vi "Get All API Interface Info.vi"(8 "error in (no error)":errorcluster, 11 "CSM-Helper in":refnum<class "CSM-Helper.lvclass">) -> (0 "error out":errorcluster, 2 "Array":cluster{string, "Array":T1[], "Response":T1[]}[](array[cluster]), 3 "CSM-Helper out":refnum<class "CSM-Helper.lvclass">)   [LabVIEW 2017, in "CSM-Helper.lvclass"]
doc: "### Get All API Interface Info.vi\n\n-- <b>Controls</b> --\n- <b>CSM-Helper in</b>: CSMHelper input\n\n-- <b>Indicators</b> --\n- <b>Array</b>:\n- <b>CSM-Helper out</b>: CSMHelper output"
uses:
  CSM-Helper.lvclass
  Typedef/Def-Argument Info.ctl
  Get Interface Info.vi
  Properties/Read APIs.vi
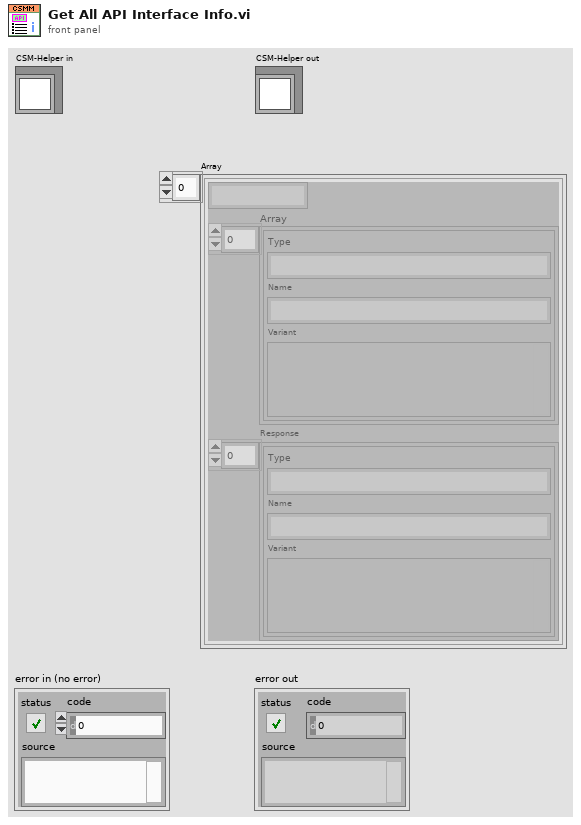
[diagram p1: front panel]
types:
  T1 = typedef "CSM-Helper.lvclass/Def-Argument Info.ctl" = cluster{"Type":string, "Name":string, "Variant":variant}
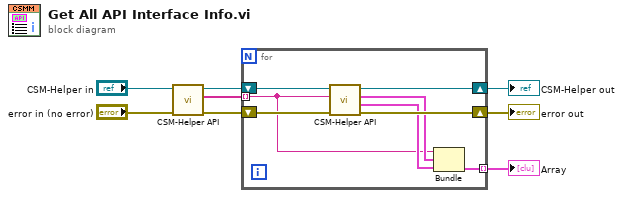
[diagram p0: block diagram]
diagram:
  n1 = call-poly "CSM-Helper API.vi"("error in (no error)"="error in (no error)", "CSM-Helper in"="CSM-Helper in") -> ("error out"=w2:errorcluster, "Value"=w5:string[], "CSM-Helper out"=w3:refnum<class "CSM-Helper.lvclass">)  [unwired: 7 in]
  n2 = for {
    shift-right: [w14] -> w6
    shift-left: w2 -> [w16]
    shift-right: [w15] -> w8
    shift-left: w3 -> [w10]
    tunnel: w5 -> [w9] mode=indexing
    tunnel: [w11] -> w4 mode=indexing
    n3 = call-poly "CSM-Helper API.vi"("error in (no error)"=w16, "CASE"=w9, "CSM-Helper in"=w10) -> ("error out"=w14:errorcluster, "Response"=w13:T1[], "Array"=w12:T1[], "CSM-Helper out"=w15:refnum<class "CSM-Helper.lvclass">)  [unwired: 5 in]
    n4 = Bundle(w9, "Array"=w12, "Response"=w13) -> (w11:cluster{string, "Array":T1[], "Response":T1[]})  [unwired: 1 in]
  }
  "CSM-Helper out" <- w8
  "error out" <- w6
  "Array" <- w4
